vi "Reserve (1 Session).vi"(6 "timeout in milliseconds":i32, 8 "error in":errorcluster, 9 "instrument type ID":string, 10 "pin or relay names":string[](array[string]), 11 "Measurement Context In":refnum<class "MeasurementContext.lvclass">) -> (0 "error out":errorcluster, 1 "gRPC clients out":T1, 2 "session information":T3, 3 "Measurement Context out":refnum<class "MeasurementContext.lvclass">)   [LabVIEW 2021, in "Measurement Service Helpers.lvlib"]
doc: "Reserves a single session based on the provided pin information. In the event that the pin information corresponds to multiple sessions, this VI will throw an error."
uses:
  Measurement Service Helpers.lvlib
  <vilib>/MeasurementLink/MeasurementLink Session Management Client/RPC Messages/ni_measurementlink_sessionmanagement_v1_SessionInformation.ctl
  <vilib>/MeasurementLink/MeasurementLink Session Management Client/RPC Messages/nidevice_grpc_Session.ctl
  <vilib>/MeasurementLink/MeasurementLink Session Management Client/RPC Messages/ni_measurementlink_sessionmanagement_v1_ChannelMapping.ctl
  GRPC Clients.ctl
  <vilib>/gRPC/LabVIEW gRPC Library/Shared/grpcId.ctl
  <vilib>/MeasurementLink/MeasurementLink Measurement Server/Classes/MeasurementContext/MeasurementContext.lvclass
  <vilib>/MeasurementLink/MeasurementLink Session Management Client/MeasurementLink Session Management Client.lvlib
  <vilib>/gRPC/LabVIEW gRPC Library/grpc-lvsupport-release.lvlib
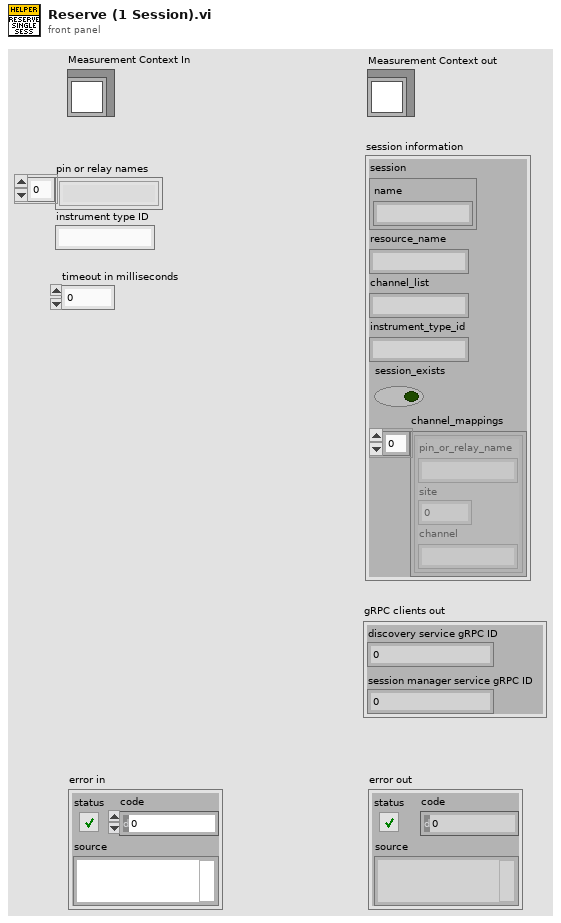
[diagram p1: front panel]
types:
  T1 = typedef "Measurement Service Helpers.lvlib/GRPC Clients.ctl" = cluster{"discovery service gRPC ID":T2, "session manager service gRPC ID":T2}
  T2 = typedef "grpc-lvsupport-release.lvlib/grpcId.ctl" = u64
  T3 = typedef "MeasurementLink Session Management Client.lvlib/ni_measurementlink_sessionmanagement_v1_SessionInformation.ctl" = cluster{"session":T4, "resource_name":string, "channel_list":string, "instrument_type_id":string, "session_exists":bool, "channel_mappings":T5[]}
  T4 = typedef "MeasurementLink Session Management Client.lvlib/nidevice_grpc_Session.ctl" = cluster{"name":string}
  T5 = typedef "MeasurementLink Session Management Client.lvlib/ni_measurementlink_sessionmanagement_v1_ChannelMapping.ctl" = cluster{"pin_or_relay_name":string, "site":i32, "channel":string}
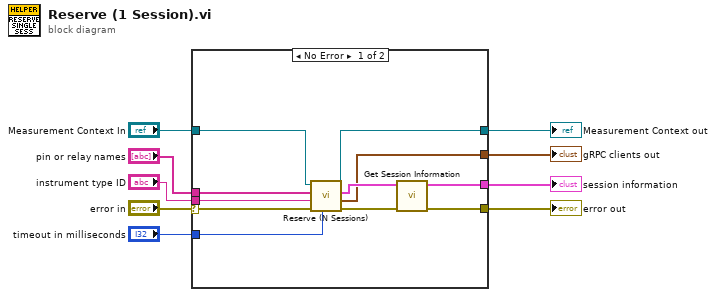
[diagram p0: block diagram]
diagram:
  n1 = case shown="No Error" "error in" {
    selector: "error in" -> [w11 w22]
    tunnel: [w20 w22] -> w9
    tunnel: [w19 _] -> w8
    tunnel: "Measurement Context In" -> [w17 w21]
    tunnel: [w16 w21] -> w6
    tunnel: "pin or relay names" -> [w15 _]
    tunnel: "instrument type ID" -> [w14 _]
    tunnel: "timeout in milliseconds" -> [w13 _]
    tunnel: [w10 _] -> w1
    frame No Error {
      n2 = call "Reserve (N Sessions).vi"("timeout in milliseconds"=w13, "error in"=w11, "instrument type ID"=w14, "pin or relay names"=w15, "Measurement Context In"=w17) -> ("error out"=w18:errorcluster, "gRPC clients out"=w10:T1, "session information"=w12:T3[], "Measurement Context out"=w16:refnum<class "MeasurementContext.lvclass">)  [unwired: 3 in]
      n3 = call "Get Session Information.vi"("error in (no error)"=w18, "session information"=w12) -> ("error out"=w20:errorcluster, "session information"=w19:T3)  [unwired: 8 in]
    }
    frame Error {
    }
  }
  "error out" <- w9
  "session information" <- w8
  "gRPC clients out" <- w1
  "Measurement Context out" <- w6
